vi "CLD 7 Time Stamp to Initialization String exercise.vi"(8 "Error In":errorcluster) -> (0 "Error Out":errorcluster, 3 "Code String Out":string)   [LabVIEW 2020]
doc: "CLD 7 exercise"
panel:
  in  "Weekday":string[](array[string])=["Sun", "Mon", "Tue", "Wed", "Thu", "Fri"]
  out "%Z string":string
  out "%z string":string
  out "%X string":string
  out "%x string":string
  out "%u string":string
  out "%c string":string
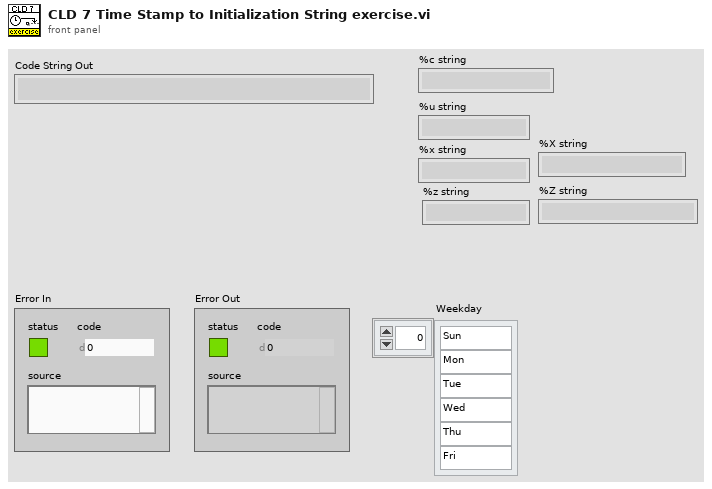
[diagram p1: front panel]
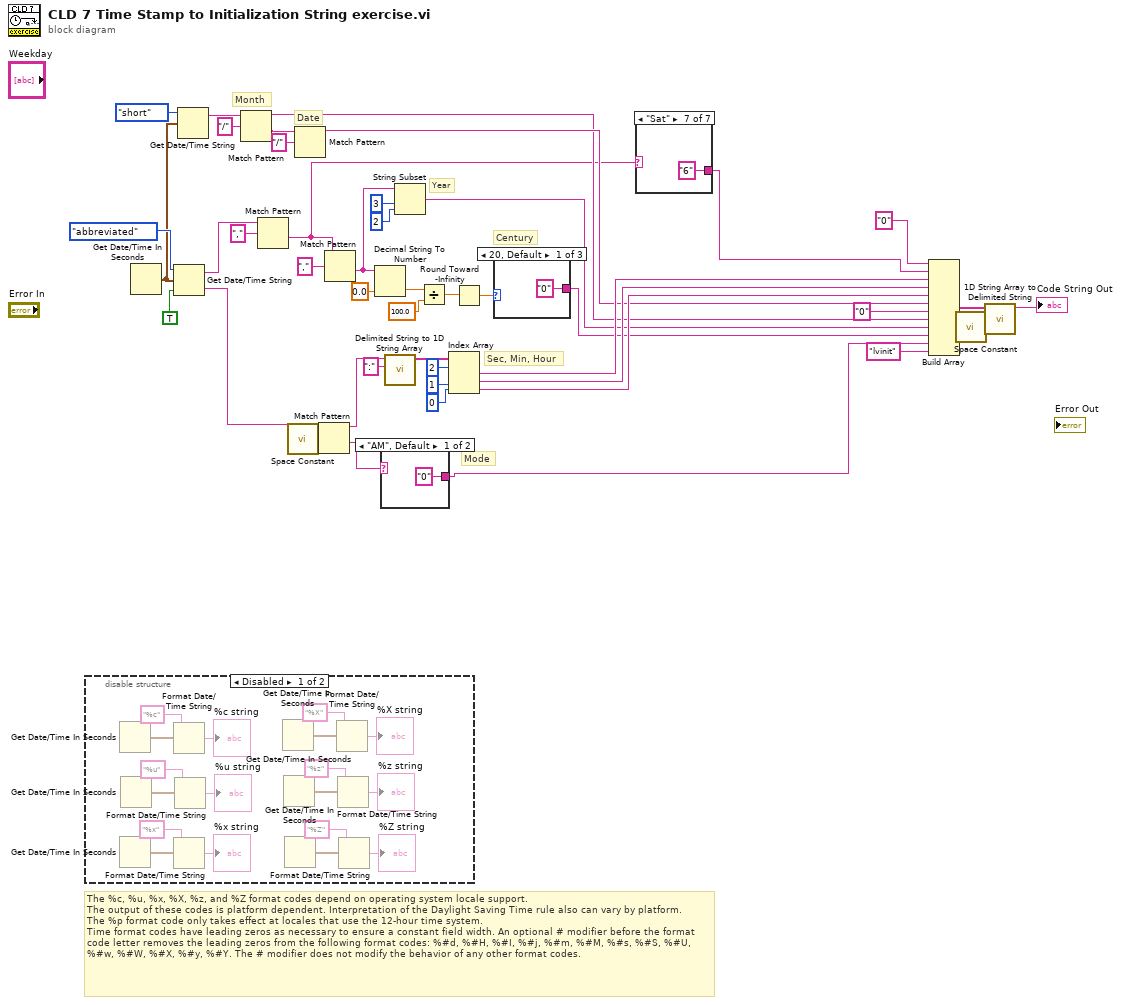
[diagram p0: block diagram]
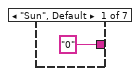
[diagram p2: hidden frame]
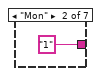
[diagram p3: hidden frame]
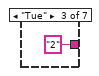
[diagram p4: hidden frame]
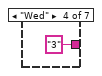
[diagram p5: hidden frame]
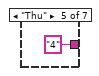
[diagram p6: hidden frame]
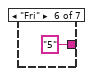
[diagram p7: hidden frame]
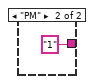
[diagram p8: hidden frame]
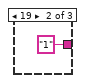
[diagram p9: hidden frame]
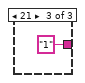
[diagram p10: hidden frame]
diagram:
  # "Date"
  # "Month"
  # "Year"
  # "Century"
  # "Mode"
  # "Sec, Min, Hour"
  # "The %c, %u, %x, %X, %z, and %Z format codes depend on operating system locale support. \nThe output of these codes is platform dependent. Interpretation of the Daylight Saving Time rule also can vary by platform. \nThe %p format code only takes effect at locales that use the 12-hour time system. \nTime format codes have leading zeros as necessary to ensure a constant field width. An optional # modifier before the format code letter removes the leading zeros from the following format codes: %#d, %#H, %#I, %#j, %#m, %#M, %#s, %#S, %#U, %#w, %#W, %#X, %#y, %#Y. The # modifier does not modify the behavior of any other format codes."
  n1 = disable-structure shown="Disabled" {
    frame Disabled {
      n2 = Get Date/Time In Seconds() -> (seconds since 1Jan1904=w62:timestamp)
      n3 = Get Date/Time In Seconds() -> (seconds since 1Jan1904=w60:timestamp)
      n4 = Get Date/Time In Seconds() -> (seconds since 1Jan1904=w61:timestamp)
      n5 = Format Date/Time String(time format string (%c)="%c", seconds (now)=w62) -> (date/time string=→"%c string":string)  [unwired: 1 in]
      n6 = Format Date/Time String(time format string (%c)="%x", seconds (now)=w60) -> (date/time string=→"%x string":string)  [unwired: 1 in]
      n7 = Format Date/Time String(time format string (%c)="%u", seconds (now)=w61) -> (date/time string=→"%u string":string)  [unwired: 1 in]
      n8 = Get Date/Time In Seconds() -> (seconds since 1Jan1904=w53:timestamp)
      n9 = Get Date/Time In Seconds() -> (seconds since 1Jan1904=w50:timestamp)
      n10 = Get Date/Time In Seconds() -> (seconds since 1Jan1904=w47:timestamp)
      n11 = Format Date/Time String(time format string (%c)="%X", seconds (now)=w53) -> (date/time string=→"%X string":string)  [unwired: 1 in]
      n12 = Format Date/Time String(time format string (%c)="%z", seconds (now)=w50) -> (date/time string=→"%z string":string)  [unwired: 1 in]
      n13 = Format Date/Time String(time format string (%c)="%Z", seconds (now)=w47) -> (date/time string=→"%Z string":string)  [unwired: 1 in]
    }
    frame Enabled {
    }
  }
  n14 = Get Date/Time In Seconds() -> (seconds since 1Jan1904=w29:timestamp)
  n15 = Get Date/Time String(date format (0)=enum16{"short", "long", "abbreviated"}."abbreviated", seconds (now)=w29, want seconds? (F)=TRUE) -> (date string=w40:string, time string=w42:string)
  n16 = Get Date/Time String(date format (0)=enum16{"short", "long", "abbreviated"}."short", seconds (now)=w29) -> (date string=w26:string)  [unwired: 1 in, 1 out]
  n17 = Match Pattern(string=w26, regular expression="/") -> (before substring=w10:string, after substring=w24:string)  [unwired: 1 in, 2 out]
  n18 = Match Pattern(string=w40, regular expression=",") -> (after substring=w2:string)  [unwired: 1 in, 3 out]
  n19 = call <vilib>:"Space Constant.vi"() -> ("String"=w39:string)
  n20 = Match Pattern(string=w24, regular expression="/") -> (before substring=w12:string)  [unwired: 1 in, 3 out]
  n21 = Match Pattern(string=w42, regular expression=w39) -> (before substring=w23:string, after substring=w17:string)  [unwired: 1 in, 2 out]
  n22 = Match Pattern(string=w2, regular expression=",") -> (after substring=w32:string)  [unwired: 1 in, 3 out]
  n23 = Decimal String To Number(string=w32, default (0L)=0.0 ("default (0 I32)")) -> (number=w36:dbl)  [unwired: 1 in, 1 out]
  n24 = case shown="\"AM\", Default" w17 {
    tunnel: ["0" ("string") "1" ("string")] -> w7
    frame "AM", Default {
    }
    frame "PM" {
    }
  }
  n25 = call <vilib>:"Delimited String to 1D String Array.vi"("delimiter"=":", "delimited string"=w23) -> ("string array"=w21:string[])  [unwired: 9 in]
  n26 = String Subset(string=w32, offset (0)=3, length (rest)=2 ("length (rest)")) -> (substring=w9:string)
  n27 = Divide(x=w36, y=100.0) -> (x/y=w33:dbl)
  n28 = Index Array(array=w21, index #1=2 ("index"), index #2=1 ("index"), index #3=0 ("index")) -> (element #1=w15:string, element #2=w14:string, element #3=w13:string)
  n29 = Round Toward -Infinity(1:w33) -> (0:w34:dbl)
  n30 = case shown="20, Default" w34 {
    tunnel: ["0" ("string") "1" ("string") "1" ("string")] -> w8
    frame 20, Default {
    }
    frame 19 {
    }
    frame 21 {
    }
  }
  n31 = case shown="\"Sat\"" w2 {
    tunnel: ["0" "1" "2" "3" "4" "5" "6"] -> w1
    frame "Sun", Default {
    }
    frame "Mon" {
    }
    frame "Tue" {
    }
    frame "Wed" {
    }
    frame "Thu" {
    }
    frame "Fri" {
    }
    frame "Sat" {
    }
  }
  n32 = Build Array("0" ("string"), w1, w15, w14, w13, w12, "0" ("string"), w10, w9, w8, w7, "lvinit" ("string")) -> (w5:string[])
  n33 = call <vilib>:"Space Constant.vi"() -> ("String"=w4:string)
  n34 = call <vilib>:"1D String Array to Delimited String.vi"("delimiter"=w4, "string array"=w5) -> ("delimited string"=→"Code String Out":string)  [unwired: 9 in]
